vi "SGUI Set Control Enabled State By Label.vi"(6 "error in":errorcluster, 8 "labels (empty)":string, 9 "Enabled? (False)":bool) -> (7 "error out":errorcluster, 11 "control references out":refnum<vi>[](array[refnum]))   [LabVIEW 2013, in "varilib.lvlib"]
doc: "This VI sets enabled state of control(s) designated by label(s) name string. Multiple can be set at once by using multiline string for both 'labels'. One line per control. Enabled? set to False sets Disabled state to 'Disabled and grayed'.\n\nThi VI ignores input errors (will execute anyway) however will generate error if any of the named controls is not found or writting to it fails (invalid type of control)."
uses:
  varilib.lvlib
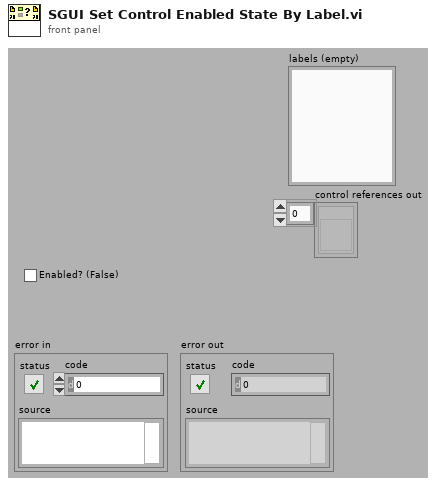
[diagram p1: front panel]
types:
  T1 = enum8{"Enabled", "Disabled", "Disabled and Grayed Out"}
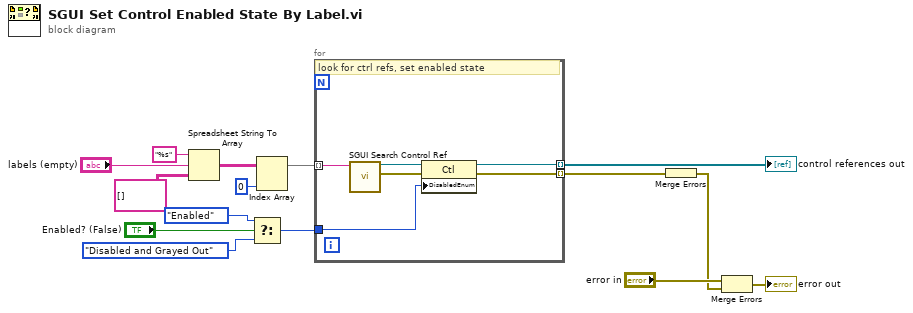
[diagram p0: block diagram]
diagram:
  n1 = Spreadsheet String To Array(format string="%s", spreadsheet string="labels (empty)", array type (2D Dbl)=string[][] []) -> (array=w15:string[][])  [unwired: 1 in]
  n2 = Select(t=T1."Enabled" ("Disabled"), s="Enabled? (False)", f=T1."Disabled and Grayed Out" ("Disabled")) -> (s? t:f=w4:T1)
  n3 = Index Array(array=w15, index (col)=0 ("disabled index (col)")) -> (element=w2:string[])  [unwired: 1 in]
  n4 = for {
    tunnel: w2 -> [w21] mode=indexing
    tunnel: [w17] -> w13 mode=indexing
    tunnel: [w18] -> w14 mode=indexing
    tunnel: w4 -> [w16]
    # "look for ctrl refs, set enabled state"
    n5 = call "SGUI Search Control Ref.vi"("control label (empty)"=w21) -> ("error out"=w20:errorcluster, "control ref out"=w19:refnum<vi>)  [unwired: 8 in, 1 out]
    n6 = property class="Ctl"(reference=w19, error in=w20, "DisabledEnum"=w16) -> (reference out=w17:refnum<vi>, error out=w18:errorcluster)
  }
  "control references out" <- w13
  n7 = Merge Errors(w14) -> (w9:errorcluster)
  n8 = Merge Errors("error in", w9) -> (→"error out":errorcluster)
